vi "BMark_OpenWindow.vi"(8 "error in (no error)":errorcluster, 11 "Bookmark manager window reference":refnum<vi>) -> (0 "error out":errorcluster, 2 "bounds":T1, 3 "Bookmark manager window reference out":refnum<vi>)   [LabVIEW 2017]
uses:
  <resource>/dialog/lvconfig.llb/LV Config Read String.vi
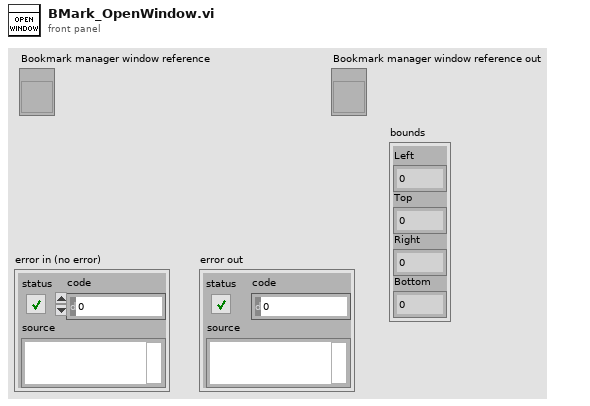
[diagram p1: front panel]
types:
  T1 = cluster{"Left":i16, "Top":i16, "Right":i16, "Bottom":i16}
  T2 = enum32{"Invalid", "Standard", "Closed", "Hidden", "Minimized", "Maximized"}
  T3 = typedef "LVAllMonitorsDisplayTypeDef.ctl" = cluster{"Bounds":cluster{"Left":i16, "Top":i16, "Right":i16, "Bottom":i16}, "Depth":i16}[]
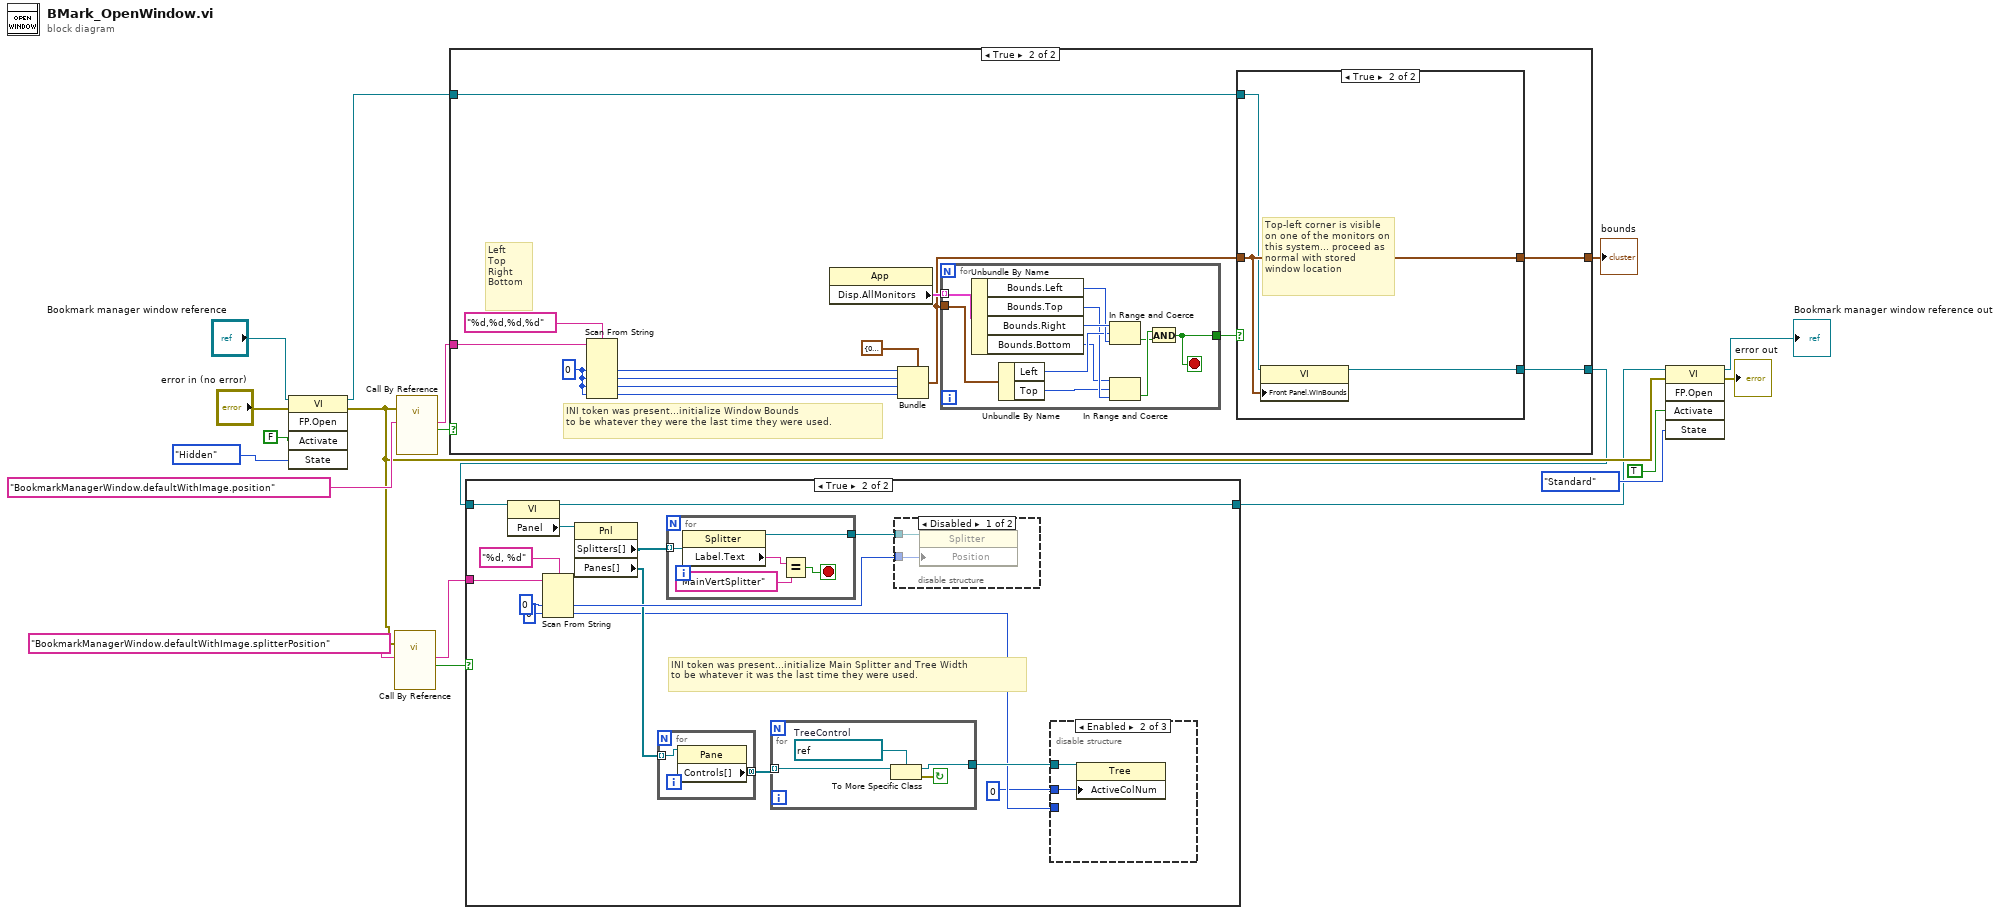
[diagram p0: block diagram]
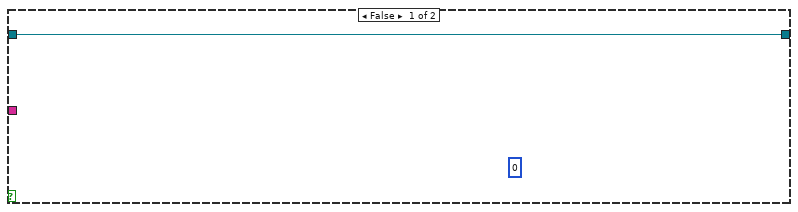
[diagram p2: hidden frame]
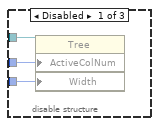
[diagram p4: hidden frame]
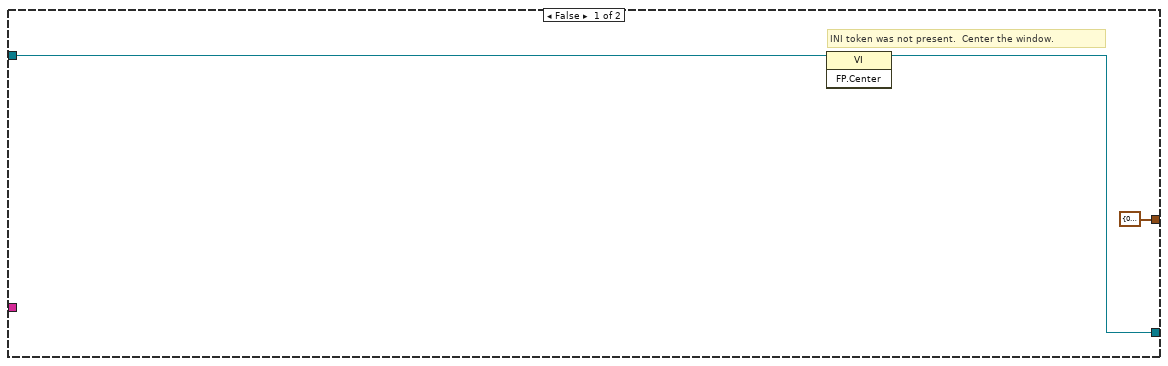
[diagram p6: hidden frame]
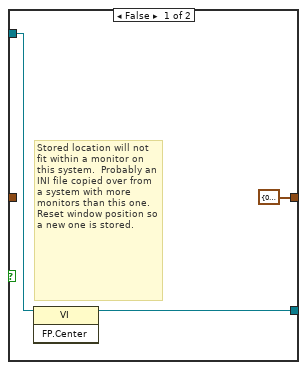
[diagram p7: hidden frame]
diagram:
  n1 = invoke class="VI" method="FP.Open"(reference="Bookmark manager window reference", error in="error in (no error)", "Activate"=FALSE ("Activate?"), "State"=T2."Hidden") -> (reference out=w3:refnum<vi>, error out=w6:errorcluster)  [unwired: 1 in, 3 out]
  n2 = call-by-ref "?"(error in=w6, "key"="BookmarkManagerWindow.defaultWithImage.splitterPosition") -> ("found?"=w5:bool, "value"=w4:string)  [unwired: 5 in, 3 out]
  n3 = call-by-ref "?"(error in=w6, "key"="BookmarkManagerWindow.defaultWithImage.position") -> ("found?"=w11:bool, "value"=w13:string)  [unwired: 5 in, 3 out]
  n4 = case shown="True" w11 {
    tunnel: [T1 {"Left"=0, "Top"=0, "Right"=0, "Bottom"=0} ("Front Panel.PanelBounds") w25] -> w8
    tunnel: w13 -> [_ w36]
    tunnel: w3 -> [w21 w24]
    tunnel: [w20 w23] -> w2
    frame False {
      # "INI token was not present.  Center the window."
      n5 = invoke class="VI" method="FP.Center"(reference=w21) -> (reference out=w20:refnum<vi>)  [unwired: 2 in, 2 out]
    }
    frame True {
      w34 = i16 0 ("default value 1")
      # "Left\nTop\nRight\nBottom"
      # "INI token was present...initialize Window Bounds\nto be whatever they were the last time they were used."
      n6 = Scan From String(format string="%d,%d,%d,%d", input string=w36, default 1=w34, default 2=w34, default 3=w34, default 4=w34) -> (output 1=w33:i16, output 2=w32:i16, output 3=w31:i16, output 4=w30:i16)  [unwired: 2 in, 3 out]
      n7 = property class="App"() -> ("Disp.AllMonitors"=w28:T3)  [unwired: 2 in, 2 out]
      n8 = Bundle(cluster=T1 {"Left"=0, "Top"=0, "Right"=0, "Bottom"=0} ("Front Panel.PanelBounds"), "Left"=w33, "Top"=w32, "Right"=w31, "Bottom"=w30) -> (w27:T1)
      n9 = for {
        tunnel: w28 -> [w53] mode=indexing
        tunnel: w27 -> [w52]
        tunnel: [w43] -> w26
        stop <- w43 stop-if-true
        n10 = Unbundle By Name(w53) -> ("Bounds.Left"=w50:i16, "Bounds.Top"=w48:i16, "Bounds.Right"=w51:i16, "Bounds.Bottom"=w47:i16)
        n11 = Unbundle By Name(w52) -> ("Left"=w49:i16, "Top"=w46:i16)
        n12 = In Range and Coerce(upper limit=w51, x=w49, lower limit=w50) -> (In Range?=w44:bool)  [unwired: 1 out]
        n13 = In Range and Coerce(upper limit=w47, x=w46, lower limit=w48) -> (In Range?=w45:bool)  [unwired: 1 out]
        n14 = And(x=w45, y=w44) -> (x .and. y?=w43:bool)
      }
      n15 = case shown="True" w26 {
        tunnel: w27 -> [_ w42]
        tunnel: [T1 {"Left"=0, "Top"=0, "Right"=0, "Bottom"=0} ("Front Panel.PanelBounds") w42] -> w25
        tunnel: w24 -> [w38 w41]
        tunnel: [w37 w40] -> w23
        frame False {
          # "Stored location will not fit within a monitor on this system.  Probably an INI file copied over from a system with more monitors than this one.  Reset window position so a new one is stored."
          n16 = invoke class="VI" method="FP.Center"(reference=w38) -> (reference out=w37:refnum<vi>)  [unwired: 2 in, 2 out]
        }
        frame True {
          # "Top-left corner is visible on one of the monitors on this system... proceed as normal with stored window location"
          n17 = property class="VI"(reference=w41, "Front Panel.WinBounds"=w42) -> (reference out=w40:refnum<vi>)  [unwired: 1 in, 1 out]
        }
      }
    }
  }
  "bounds" <- w8
  n18 = case shown="True" w5 {
    tunnel: w4 -> [_ w69]
    tunnel: w2 -> [w54 w64]
    tunnel: [w54 w61] -> w1
    frame False {
      (unwired) 0 ("default value 1")
      # "INI token was not present.  Leave splitter at default"
    }
    frame True {
      # "INI token was present...initialize Main Splitter and Tree Width\nto be whatever it was the last time they were used."
      n19 = property class="VI"(reference=w64) -> (reference out=w61:refnum<vi>, "Panel"=w63:refnum<vi>)  [unwired: 1 in, 1 out]
      n20 = Scan From String(format string="%d, %d", input string=w69, default 1=0 ("default value 1"), default 2=u32 0 ("default value 2")) -> (output 1=w62:i32, output 2=w56:u32)  [unwired: 2 in, 3 out]
      n21 = property class="Pnl"(reference=w63) -> ("Splitters[]"=w65:refnum<vi>[], "Panes[]"=w58:refnum<vi>[])  [unwired: 1 in, 2 out]
      n22 = for {
        tunnel: w58 -> [w78] mode=indexing
        tunnel: [w77] -> w60 mode=concatenating
        n23 = property class="Pane"(reference=w78) -> ("Controls[]"=w77:refnum<vi>[])  [unwired: 1 in, 2 out]
      }
      n24 = for {
        tunnel: w65 -> [w87] mode=indexing
        tunnel: [w84] -> w66
        stop <- w83 stop-if-true
        n25 = property class="Splitter"(reference=w87) -> (reference out=w84:refnum<vi>, "Label.Text"=w86:string)  [unwired: 1 in, 1 out]
        n26 = Equal?(x=w86, y="MainVertSplitter") -> (x = y?=w83:bool)
      }
      n27 = for {
        tunnel: [w81] -> w59
        tunnel: w60 -> [w80] mode=indexing
        stop <- w79 continue-if-true
        w82 = refnum<vi> refnum  # TreeControl
        n28 = To More Specific Class(target class=w82, reference=w80) -> (specific class reference=w81:refnum<vi>, error out=w79:errorcluster)  [unwired: 1 in]
      }
      n29 = disable-structure shown="Disabled" {
        disable-tunnel: w66 -> [w71 _]
        disable-tunnel: w62 -> [w70 _]
        frame Disabled {
          n30 = property class="Splitter"(reference=w71, "Position"=w70) -> ()  [unwired: 1 in, 2 out]
        }
        frame Enabled {
        }
      }
      n31 = disable-structure shown="Enabled" {
        disable-tunnel: w59 -> [w74 w76 _]
        disable-tunnel: w56 -> [w73 _ _]
        disable-tunnel: 0 ("Active Cell:Active Column Number") -> [w72 w75 _]
        frame Disabled {
          n32 = property class="Tree"(reference=w74, "ActiveColNum"=w72, "Width"=w73) -> ()  [unwired: 1 in, 2 out]
        }
        frame Enabled {
          n33 = property class="Tree"(reference=w76, "ActiveColNum"=w75) -> ()  [unwired: 1 in, 2 out]
        }
        frame Disabled {
        }
      }
    }
  }
  n34 = invoke class="VI" method="FP.Open"(reference=w1, error in=w6, "Activate"=TRUE ("Activate?"), "State"=T2."Standard") -> (reference out=→"Bookmark manager window reference out":refnum<vi>, error out=→"error out":errorcluster)  [unwired: 1 in, 3 out]
